vi "Connect.vi"(8 "error in (no error)":errorcluster, 9 "timeout":i32=-1, 11 "Network Stream in":refnum<class "Network Stream Listener.lvclass">) -> (0 "error out":errorcluster, 3 "Network Stream out":refnum<class "Network Stream Listener.lvclass">)   [LabVIEW 2020, in "Network Stream Listener.lvclass"]
doc: "This method waits for a remote connection from a Network Stream Initiator."
uses:
  <vilib>/NI/Actors/Network Endpoint Actors/Protocols/Network Stream Strategy/Netowrk Stream Listener/Network Stream Listener.lvclass
  C:/Program Files (x86)/National Instruments/LabVIEW 2020/vi.lib/NI/Actors/Network Endpoint Actors/Protocols/Network Stream Strategy/Network Stream/Network Stream.lvclass
  <vilib>/NI/Actors/Network Endpoint Actors/Protocols/Network Stream Strategy/Network Stream/Network Stream.lvclass/Network Stream.ctl
  <vilib>/NI/Actors/Network Endpoint Actors/Protocols/Network Stream Strategy/Network Stream/Network Stream.lvclass
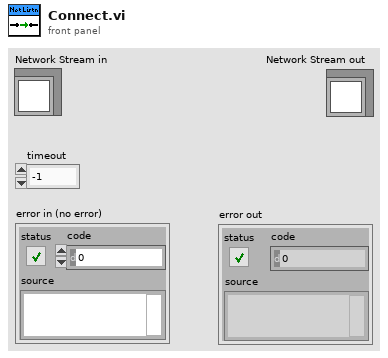
[diagram p1: front panel]
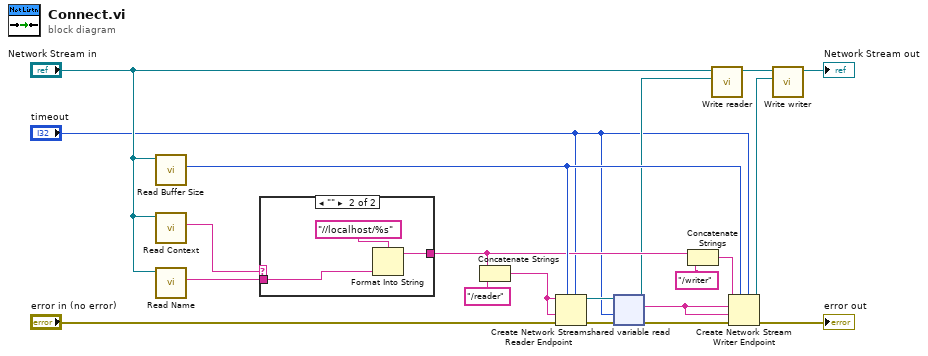
[diagram p0: block diagram]
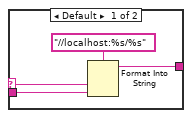
[diagram p2: hidden frame]
diagram:
  n1 = call <vilib>:"Read Buffer Size.vi"("Network Stream in"="Network Stream in") -> ("Buffer Size"=w10:i32)  [unwired: 10 in]
  n2 = call <vilib>:"Read Context.vi"("Network Stream in"="Network Stream in") -> ("Context"=w12:string)  [unwired: 10 in]
  n3 = call <vilib>:"Read Name.vi"("Network Stream in"="Network Stream in") -> ("Name"=w11:string)  [unwired: 10 in]
  n4 = case shown="\"\"" w12 {
    selector: w12 -> [w21 _]
    tunnel: [w23 w26] -> w7
    tunnel: w11 -> [w22 w25]
    frame Default {
      n5 = Format Into String(format string="//localhost:%s/%s", w21, w22) -> (resulting string=w23:string)  [unwired: 2 in, 1 out]
    }
    frame "" {
      n6 = Format Into String(format string="//localhost/%s", w25) -> (resulting string=w26:string)  [unwired: 2 in, 1 out]
    }
  }
  n7 = Concatenate Strings(w7, "/reader" ("format string")) -> (w13:string)
  n8 = Create Network Stream Reader Endpoint(5:"timeout", 7:w10, 8:"error in (no error)", 9:w13, 11:w13) -> (0:w15:errorcluster, 3:w16:refnum<k21>)  [unwired: 2 in]
  n9 = shared-variable-read(w16, w15, "timeout") -> (w5:refnum<k21>, w17:errorcluster, w18:string)  [unwired: 1 out]
  n10 = Concatenate Strings(w7, "/writer" ("format string")) -> (w20:string)
  n11 = call <vilib>:"Write reader.vi"("reader"=w5, "Network Stream in"="Network Stream in") -> ("Network Stream out"=w3:refnum<class "Network Stream Listener.lvclass">)  [unwired: 9 in]
  n12 = Create Network Stream Writer Endpoint(5:"timeout", 7:w10, 8:w17, 9:w18, 10:w18, 11:w20) -> (0:→"error out":errorcluster, 3:w6:refnum<k21>)  [unwired: 1 in]
  n13 = call <vilib>:"Write writer.vi"("writer"=w6, "Network Stream in"=w3) -> ("Network Stream out"=→"Network Stream out":refnum<class "Network Stream Listener.lvclass">)  [unwired: 9 in]
